vi "Test2_query.vi"() -> ()   [LabVIEW 2019]
panel:
  in  "Acceleration":u16
  in  "Input Speed":i16
  in  "Target":i32
  out "Flags":T1
  in  "stop":bool
  in  "Address":u8
  out "Query Speed":i16
  out "Position":i32
  in  "COM Port for serial\nconnection. Check device\nmanager.":string
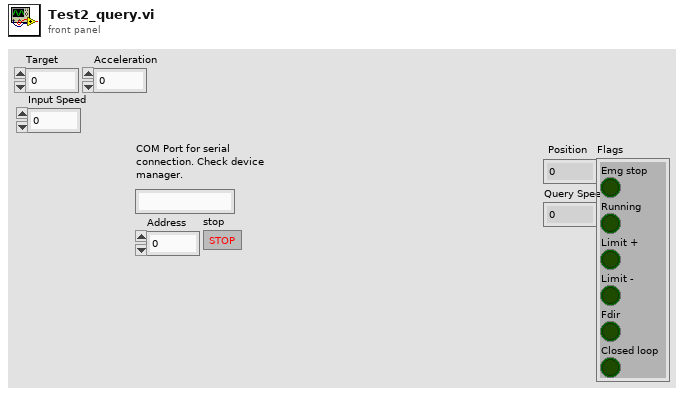
[diagram p1: front panel]
types:
  T1 = cluster{"Emg stop":bool, "Running":bool, "Limit +":bool, "Limit -":bool, "Fdir":bool, "Closed loop":bool}
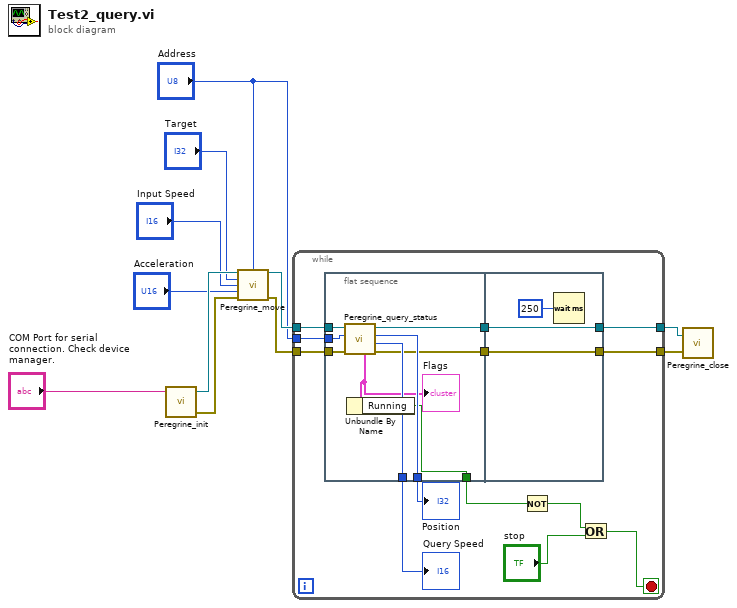
[diagram p0: block diagram]
diagram:
  n1 = call "Peregrine_init.vi"("COM Port for serial\nconnection. Check device\nmanager."="COM Port for serial\nconnection. Check device\nmanager.") -> ("error out"=w8:errorcluster, "Handle out"=w7:refnum<visa-resource-name>)  [unwired: 3 in]
  n2 = call "Peregrine_move.vi"("Handle in"=w7, "Address"="Address", "Target"="Target", "Speed"="Input Speed", "Acceleration"="Acceleration", "error"=w8) -> ("Handle out"=w6:refnum<visa-resource-name>, "error out"=w5:errorcluster)  [unwired: 8 in]
  n3 = while {
    tunnel: "Address" -> [w23]
    tunnel: w5 -> [w24]
    tunnel: w6 -> [w22]
    tunnel: [w18] -> w10
    tunnel: [w16] -> w9
    stop <- w14 stop-if-true
    n4 = flat-sequence {
      tunnel: w24 -> [w33]
      tunnel: w23 -> [w32]
      tunnel: w22 -> [w31]
      tunnel: [w30] -> w21
      tunnel: [w29] -> w20
      tunnel: [w28] -> w19
      tunnel: [w27] -> w17
      tunnel: [w25] -> w13
      tunnel: w19 -> [w35]
      tunnel: [w35] -> w18
      tunnel: w17 -> [w34]
      tunnel: [w34] -> w16
      frame #0 {
        n5 = call "Peregrine_query_status.vi"("error"=w33, "Address"=w32, "Handle in"=w31) -> ("error out"=w28:errorcluster, "Speed"=w30:i16, "Position"=w29:i32, "Handle out"=w27:refnum<visa-resource-name>, "Flags"=w26:T1)  [unwired: 4 in]
        "Flags" <- w26
        n6 = Unbundle By Name(w26) -> ("Running"=w25:bool)
      }
      frame #1 {
        n7 = Wait (ms)(milliseconds to wait=u32 250) -> ()  [unwired: 1 out]
      }
    }
    n8 = Not(x=w13) -> (.not. x?=w12:bool)
    n9 = Or(x=w12, y="stop") -> (x .or. y?=w14:bool)
    "Position" <- w20
    "Query Speed" <- w21
  }
  n10 = call "Peregrine_close.vi"("error in (no error)"=w10, "Handle in"=w9) -> ()  [unwired: 1 in, 1 out]
